vi "2.vi"() -> ()   [LabVIEW 2017]
panel:
  out "Array 2":bool[](array[boolean])
  in  "Array":bool[](array[boolean])
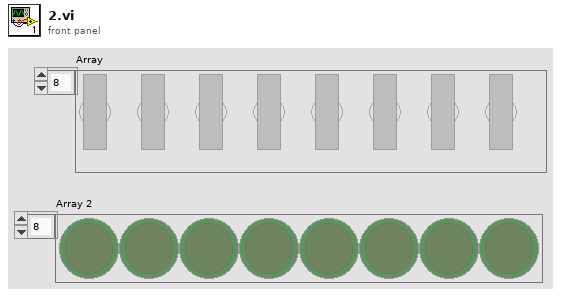
[diagram p1: front panel]
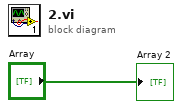
[diagram p0: block diagram]
diagram:
  "Array 2" <- "Array"
